vi "NIMS_DF_iir_lpnormconstr.vi"(0 "n":i32, 1 "e":dbl[](array[numeric]), 2 "w":dbl[](array[numeric]), 3 "p":i32=128, 5 "d":i32=1, 9 "f":dbl[](array[numeric]), 12 "mag":dbl[](array[numeric]), 13 "r":dbl=0.9999) -> (4 "b":dbl[](array[numeric]), 6 "a":dbl[](array[numeric]), 8 "err":dbl=0.9999, 10 "SOS":dbl[][](array[numeric]), 14 "error":i32, 15 "gain":dbl=0.9999)   [LabVIEW 2017, in "NI_DigFilter_MathScript.lvlib"]
uses:
  <vilib>/addons/Digital Filter Design/NI_DigFilter_MathScript.lvlib
  <vilib>/addons/Digital Filter Design/_LpNorm.llb/dfd_Lp Norm Filter Type.ctl
  <vilib>/addons/Digital Filter Design/Design.llb/DFD Least Pth Norm Design by Newton.vi
  <vilib>/addons/Digital Filter Design/NI_DigFilterLicensed.lvlib
panel:
  in  "reserved3":dbl[](array[numeric])
  in  "reserved2":dbl[](array[numeric])
  in  "reserved1":dbl=nan
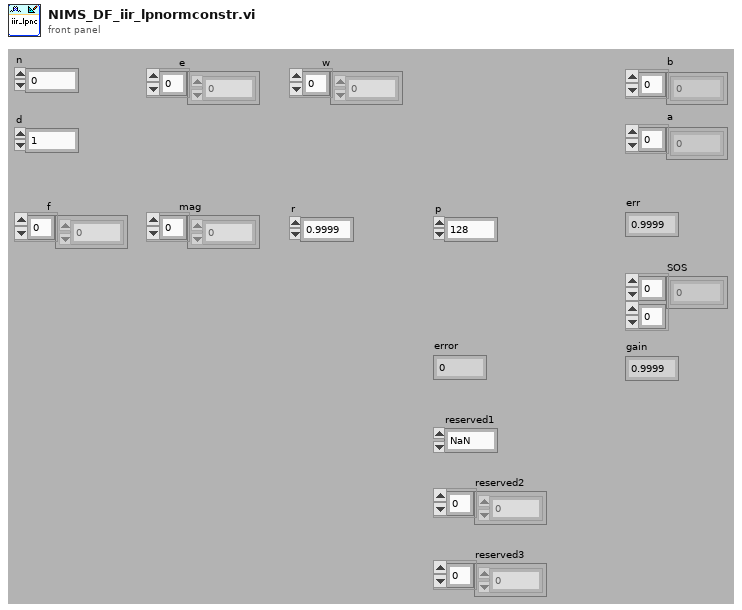
[diagram p1: front panel]
types:
  T1 = typedef "NI_DigFilterLicensed.lvlib/dfd_Lp Norm Filter Type.ctl" = enum16{"Symmetric", "Antisymmetric", "Differentiator", "Hilbert", "Minimum Phase", "Maximum Phase"}
  T2 = cluster{"frequency point":cluster{"frequency":dbl, "magnitude":dbl, "weight":dbl, "phase":dbl}[]}[]
  T3 = typedef "NI_DigFilterLicensed.lvlib/DFD Filter Obj.ctl" = cluster{"mSRate_Fs":dbl, "mSRate_Version":string, "mSRate_Comments":string, "mSRate_OrgCoef":T4, "mSRate_CurCoef":T4, "mSRate_Quantized?":bool, "mSRate_QCoef":T4, "mSRate_QSettings":T6[], "mSRate_Order":i32, "mSRate_Scaling":cluster{"mSRate_ScaleByPowerOf2?":bool, "mSRate_ScaleType":T8}}
  T4 = typedef "NI_DigFilterLicensed.lvlib/DFD Filter Coef.ctl" = cluster{"type":T5, "gain":dbl, "coef a (k)":dbl[], "coef b (v)":dbl[]}
  T5 = typedef "NI_DigFilterLicensed.lvlib/DFD Filter Structure Type Selector.ctl" = enum16{"Undefined", "FIR Direct Form", "FIR Direct Form Transposed", "FIR Symmetric", "FIR Antisymmetric", "IIR Direct Form I", "IIR Direct Form I Transposed", "IIR Direct Form II", "IIR Direct Form II Transposed", "IIR Cascaded Second Order Sections Form I", "IIR Cascaded Second Order Sections Form I Transposed", "IIR Cascaded Second Order Sections Form II", "IIR Cascaded Second Order Sections Form II Transposed", "Lattice Allpass (basic sections)", "Lattice Allpass (one multiplier sections)", "Lattice Allpass (normalized sections)", "Lattice AR (basic sections)", "Lattice AR (one multiplier sections)", "Lattice AR (normalized sections)", "Lattice MA (minimum phase)", "Lattice MA (maximum phase)", "Lattice ARMA (basic sections)", "Lattice ARMA (one multiplier sections)", "Lattice ARMA (normalized sections)"}
  T6 = typedef "NI_DigFilterLicensed.lvlib/dfd_Internal Quantization Settings.ctl" = cluster{"source":T7, "wl":i16, "iwl":i16, "overflow mode":enum16{"Saturation", "Wrap"}, "rounding mode":enum16{"Nearest", "Truncation"}, "signed?":bool}
  T7 = typedef "NI_DigFilterLicensed.lvlib/dfd_Internal Quantization Srcs.ctl" = u16
  T8 = typedef "NI_DigFilterLicensed.lvlib/DFD Coef Norm Type.ctl" = enum16{"No Norm", "Time Domain 1-Norm", "Time Domain 2-Norm", "Time Domain Inf-Norm"}
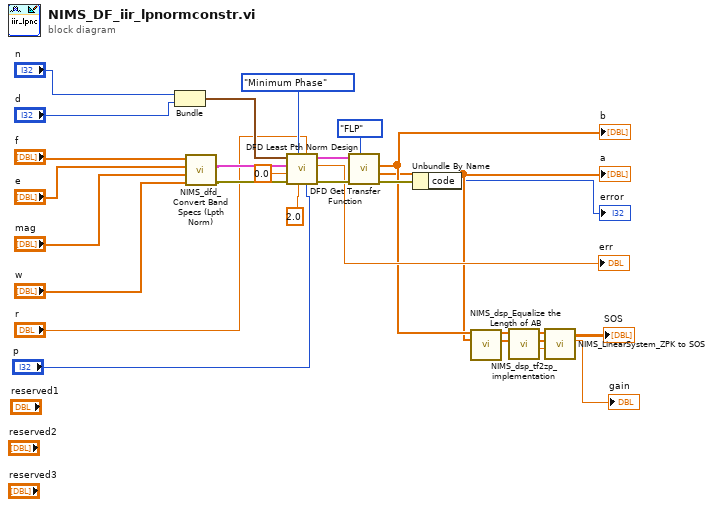
[diagram p0: block diagram]
diagram:
  n1 = Bundle("n"="n", "d"="d") -> (w15:cluster{"n":i32, "d":i32})  [unwired: 1 out]
  n2 = call <vilib>:"NIMS_dfd_Convert Band Specs (Lpth Norm).vi"("W"="w", "Amplitude"="mag", "Edges"="e", "F"="f") -> ("error out"=w18:errorcluster, "band specs"=w19:T2)  [unwired: 6 out]
  n3 = call-poly <vilib>:"DFD Least Pth Norm Design.vi"("p (128)"="p", "pole radius constraint"="r", "fs [Hz]"=2.0, "filter type"=dfd_Lp_Norm_Filter_Type."Minimum Phase", "error in (no error)"=w18, "group delay"=0.0, "band specs"=w19, "order"=w15) -> ("error out"=w23:errorcluster, "pth norm"=→"err":dbl, "filter out"=w24:T3)  [unwired: 1 out]
  n4 = call <vilib>:"DFD Get Transfer Function.vi"("type (FLP)"=enum16{"FLP", "FXP"}."FLP", "error in (no error)"=w23, "filter in"=w24) -> ("error out"=w14:errorcluster, "denominator"=w4:dbl[], "numerator"=w5:dbl[])  [unwired: 6 out]
  "b" <- w5
  "a" <- w4
  n5 = Unbundle By Name(w14) -> ("code"=→"error":i32)
  n6 = call <vilib>:"NIMS_dsp_Equalize the Length of AB.vi"("B in"=w5, "A in"=w4) -> ("B out"=w10:dbl[], "A out"=w9:dbl[])  [unwired: 12 out]
  n7 = call <vilib>:"NIMS_dsp_tf2zp_implementation.vi"("A"=w9, "B"=w10) -> ("gain"=w6:dbl, "poles"=w7:cdb[], "zeros"=w8:cdb[])  [unwired: 7 out]
  n8 = call <vilib>:"NIMS_LinearSystem_ZPK to SOS.vi"("gain"=w6, "poles"=w7, "zeros"=w8) -> ("gain"=→"gain":dbl, "SOS"=→"SOS":dbl[][])  [unwired: 3 in, 4 out]
